vi "Rcv Cmd.vi"(8 "error in":errorcluster, 11 "PAS in":refnum<class "PAS.lvclass">) -> (0 "error out":errorcluster, 3 "PAS out":refnum<class "PAS.lvclass">)   [LabVIEW 2015, in "PAS Library.lvlib" / "PAS.lvclass"]
doc: "The override of the <b>Instrument:Rcv Cmd</b> method accounts for checking for speaker switching when the object is set to autocycle. How the change in switch state is executed is left to the <b>Change Speaker State</b> command object which is sent when the state is to be changed."
uses:
  PAS.lvclass
  Instrument/Instrument.lvclass
  Switch/Switch.lvclass
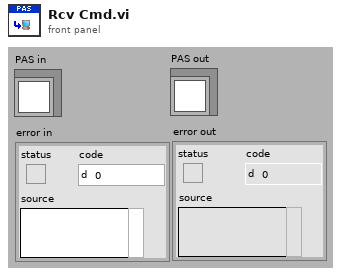
[diagram p1: front panel]
types:
  T1 = cluster{"tag":string, "section":string, "data":variant}
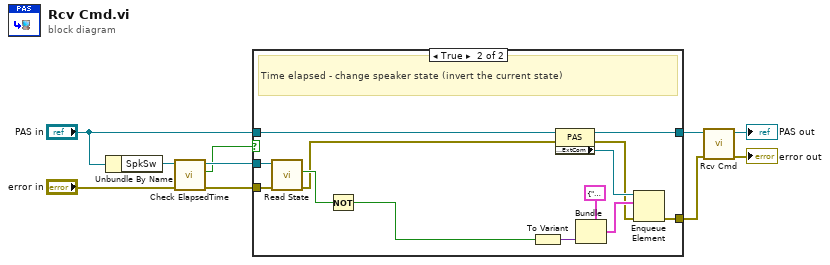
[diagram p0: block diagram]
diagram:
  n1 = Unbundle By Name("PAS in") -> ("SpkSw"=w8:refnum<class "Switch.lvclass">)
  n2 = call-dynamic "Check ElapsedTime.vi"("error in"="error in", "Switch in"=w8) -> ("error out"=w6:errorcluster, "Cycle Switch?"=w5:bool, "Switch out"=w7:refnum<class "Switch.lvclass">)  [unwired: 6 in, 1 out]
  n3 = case shown="True" w5 {
    tunnel: w7 -> [_ w25]
    tunnel: w6 -> [w11 w24]
    tunnel: "PAS in" -> [w12 w22]
    tunnel: [w12 w20] -> w3
    tunnel: [w11 w14] -> w2
    frame False {
    }
    frame True {
      # "Time elapsed - change speaker state (invert the current state)"
      n4 = call-dynamic "Read State.vi"("error in (no error)"=w24, "Switch in"=w25) -> ("error out"=w21:errorcluster, "State"=w23:bool)  [unwired: 7 in, 1 out]
      n5 = Not(x=w23) -> (.not. x?=w17:bool)
      n6 = To Variant(anything=w17) -> (Variant=w16:variant)
      n7 = property class="PAS"(reference=w22, error in=w21) -> (reference out=w20:refnum<class "PAS.lvclass">, error out=w13:errorcluster, "Accessors:ExtCom"=w19:refnum<queue>)
      n8 = Bundle(cluster=T1 {"tag"="enabled", "section"="pas.spk", "data"=variant} ("element"), "data"=w16) -> (w15:T1)  [unwired: 2 in]
      n9 = Enqueue Element(queue=w19, element=w15, error in (no error)=w13) -> (error out=w14:errorcluster)  [unwired: 1 in, 2 out]
    }
  }
  n10 = call-parent "Rcv Cmd.vi"("error in"=w2, "Instrument in"=w3) -> ("error out"=→"error out":errorcluster, "Instrument out"=→"PAS out":refnum<class "PAS.lvclass">)  [unwired: 8 in]
